vi "ApproachingStep.vi"() -> ()   [LabVIEW 2014]
uses:
  <vilib>/Platform/TimedLoop/XDataNode/timing_clust.ctl
  <vilib>/Platform/TimedLoop/XDataNode/nitl_modes.ctl
  <vilib>/Platform/TimedLoop/XDataNode/wakeup.ctl
  <vilib>/rvi/Emulation/niFpgaGetClockAttributes.vi
  <vilib>/rvi/Emulation/niFpgaSctlEmulationGetInTimedLoop.vi
  <vilib>/rvi/Emulation/niFpgaEmulationReportErrorSimple.vi
  <vilib>/rvi/eio/common/nirviEmuTemplateMethod_errors.vi
  <vilib>/rvi/Emulation/niFpgaCriticalErrorInLSC.vi
  <vilib>/Platform/TimedLoop/XDataNode/XDataNode.xnode
  <vilib>/eio/EIONode/EIONode.xnode
  <vilib>/Platform/TimedLoop/XDataNode/XDNodeRunTimeDep.lvlib
panel:
  out "ExceedUpperLimit?":bool
  out "PIZRangeExceeded?":bool
  out "Approached?":bool
  in  "stop":bool
  out "PresCurr":i16
  out "RealPIZPos":i16
  in  "RefCurr":i16
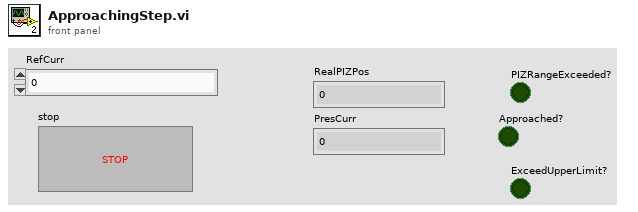
[diagram p1: front panel]
types:
  T1 = typedef "XDNodeRunTimeDep.lvlib/timing_clust.ctl" = cluster{"Expected End [f-1]":u64, "Actual End [f-1]":u64, "Finished Late? [f-1]":bool, "Expected End [i-1]":u64, "Actual End [i-1]":u64, "Finished Late? [i-1]":bool, "Expected Start [i]":u64, "Actual Start [i]":u64, "Expected Start [f]":u64, "Actual Start [f]":u64, "Source Name":string, "Structure Name":string, "Period":i64, "Deadline":i64, "Offset":i64, "Start":i64, "Priority":i32, "Timeout":i32, "Mode":T2, "Wakeup Reason":T3, "Error":errorcluster, "Source Type":string, "Secondary Source Type":string, "Global End Time":u64, "Global Start Time":u64, "Frame Duration":u64, "Iteration Duration":u64, "Assigned CPU":i32, "I/O Scan Engine Mode":u32}
  T2 = typedef "XDNodeRunTimeDep.lvlib/nitl_modes.ctl" = enum32{"No Change", "Process missed periods, maintain original phase", "Discard missed periods, maintain original phase", "Process missed periods, ignore original phase", "Discard missed periods, ignore original phase"}
  T3 = typedef "XDNodeRunTimeDep.lvlib/wakeup.ctl" = enum32{"Normal", "Aborted", "Asynchronous wakeup", "Timing source error", "Timed loop error", "Timeout"}
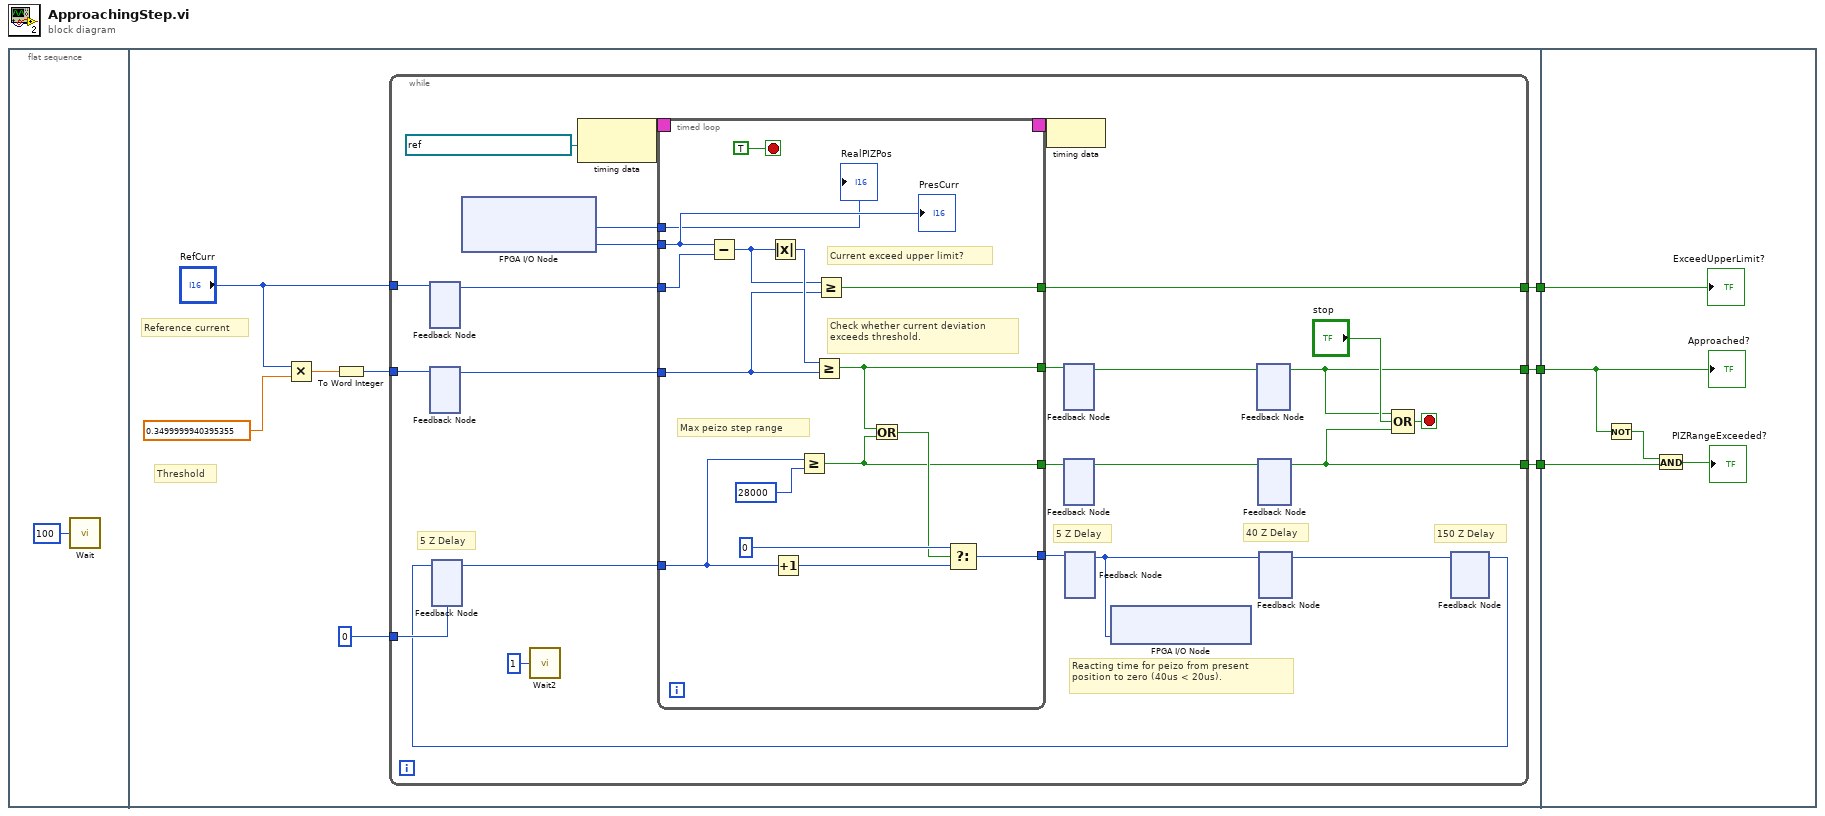
[diagram p0: block diagram]
diagram:
  n1 = flat-sequence {
    tunnel: [w9] -> w3
    tunnel: [w8] -> w2
    tunnel: [w7] -> w1
    tunnel: w3 -> [w62]
    tunnel: w2 -> [w64]
    tunnel: w1 -> [w60]
    frame #0 {
      n2 = call "Wait"("Count(uSec)"=u32 100) -> ()  [unwired: 1 out]
    }
    frame #1 {
      # "Threshold"
      # "Reference current"
      n3 = Multiply(x="RefCurr", y=sgl 0.35) -> (x*y=w6:sgl)
      n4 = To Word Integer(number=w6) -> (16bit integer=w5:i16)
      n5 = while {
        tunnel: w5 -> [w35]
        tunnel: "RefCurr" -> [w36]
        tunnel: i16 0 -> [w25]
        tunnel: [w16] -> w9
        tunnel: [w15] -> w8
        tunnel: [w14] -> w7
        stop <- w19 stop-if-true
        # "Reacting time for peizo from present \nposition to zero (40us < 20us)."
        # "150 Z Delay"
        # "40 Z Delay"
        # "5 Z Delay"
        # "5 Z Delay"
        n6 = feedback #1() -> (w31:i16)  [unwired: 1 in]
        n7 = feedback-in #1(w36) -> ()
        n8 = feedback #2() -> (w13:i16)  [unwired: 1 in]
        n9 = feedback-in #2(w35) -> ()
        n10 = feedback #3(w25) -> (w26:i16)
        n11 = xnode "FPGA I/O Node"() -> ("Connector0/AI0"=w30:i16, "Connector0/AI1"=w29:i16)  [unwired: 2 in, 2 out]
        n12 = call "Wait2"("Count(uSec)"=u32 1) -> ()  [unwired: 1 out]
        n13 = node-c288(refnum<k21> "40 MHz Onboard Clock" ("Source Name")) -> (w34:T1)
        n14 = timed-loop {
          timing: w34 -> [_]
          timing-out: [_] -> w33
          tunnel: w31 -> [w51]
          tunnel: w13 -> [w39]
          tunnel: w30 -> [w50]
          tunnel: w29 -> [w52]
          tunnel: [w41] -> w27
          tunnel: w26 -> [w43]
          tunnel: [w47] -> w28
          tunnel: [w44] -> w24
          tunnel: [w38] -> w14
          stop <- TRUE stop-if-true
          # "Current exceed upper limit?"
          # "Max peizo step range"
          # "Check whether current deviation\nexceeds threshold."
          n15 = Subtract(x=w52, y=w51) -> (x-y=w40:i16)
          n16 = Absolute Value(x=w40) -> (abs(x)=w42:i16)
          n17 = Increment(x=w43) -> (x+1=w49:i16)
          n18 = Greater Or Equal?(x=w43, y=i16 28000) -> (x >= y?=w44:bool)
          n19 = Greater Or Equal?(x=w42, y=w39) -> (x >= y?=w41:bool)
          n20 = Greater Or Equal?(x=w40, y=w39) -> (x >= y?=w38:bool)
          n21 = Or(x=w41, y=w44) -> (x .or. y?=w46:bool)
          n22 = Select(t=i16 0, s=w46, f=w49) -> (s? t:f=w47:i16)
          "RealPIZPos" <- w50
          "PresCurr" <- w52
        }
        n23 = node-c288(w33) -> ()
        n24 = feedback #4() -> (w22:bool)  [unwired: 1 in]
        n25 = feedback-in #4(w27) -> ()
        n26 = feedback #5() -> (w23:bool)  [unwired: 1 in]
        n27 = feedback-in #5(w24) -> ()
        n28 = feedback #6() -> (w21:i16)  [unwired: 1 in]
        n29 = feedback-in #6(w28) -> ()
        n30 = xnode "FPGA I/O Node"("Connector0/AO0"=w21) -> ()  [unwired: 1 in, 1 out]
        n31 = feedback #7() -> (w16:bool)  [unwired: 1 in]
        n32 = feedback-in #7(w22) -> ()
        n33 = feedback #8() -> (w15:bool)  [unwired: 1 in]
        n34 = feedback-in #8(w23) -> ()
        n35 = feedback #9() -> (w18:i16)  [unwired: 1 in]
        n36 = feedback-in #9(w21) -> ()
        n37 = Compound Arithmetic op=OR(w16, "stop", w15) -> (w19:bool)
        n38 = feedback #10() -> (w17:i16)  [unwired: 1 in]
        n39 = feedback-in #3(w17) -> ()
        n40 = feedback-in #10(w18) -> ()
      }
    }
    frame #2 {
      n41 = Not(x=w62) -> (.not. x?=w61:bool)
      n42 = And(x=w61, y=w64) -> (x .and. y?=→"PIZRangeExceeded?":bool)
      "Approached?" <- w62
      "ExceedUpperLimit?" <- w60
    }
  }
